vi "Interface_Asset_Launch Process.vi"(8 "error in (no error)":errorcluster, 10 "data value reference":refnum<data-value>, 11 "Interface_Asset in":refnum<class "Interface_Asset.lvclass">) -> ()   [LabVIEW 2015, in "Interface_Asset.lvclass"]
uses:
  Interface_Asset.lvclass
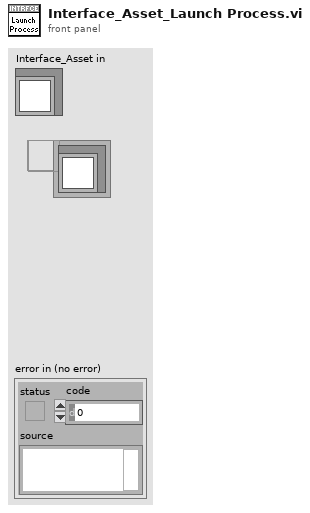
[diagram p1: front panel]
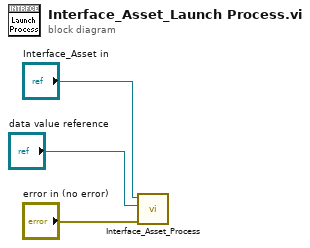
[diagram p0: block diagram]
diagram:
  n1 = call-dynamic "Interface_Asset_Process.vi"("error in (no error)"="error in (no error)", "data value reference"="data value reference", "Interface_Asset in"="Interface_Asset in") -> ()  [unwired: 9 in]
